vi "Parse Controls and Indicators.vi"(8 "Error In":errorcluster, 9 "Indicators":T1[](array[typedef]), 11 "Controls":T1[](array[typedef])) -> (0 "Error Out":errorcluster, 2 "Indicators  Wiki Syntax":string, 3 "Contorls Wiki Syntax":string)   [LabVIEW 2014]
uses:
  Control Info.ctl
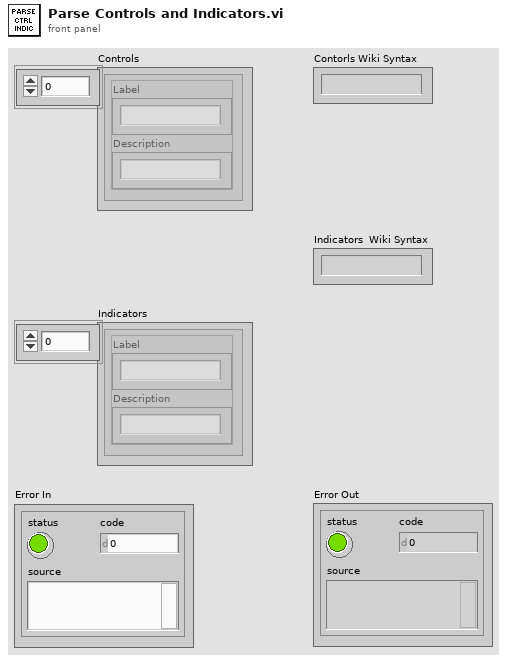
[diagram p1: front panel]
types:
  T1 = typedef "Control Info.ctl" = cluster{"Label":string, "Description":string}
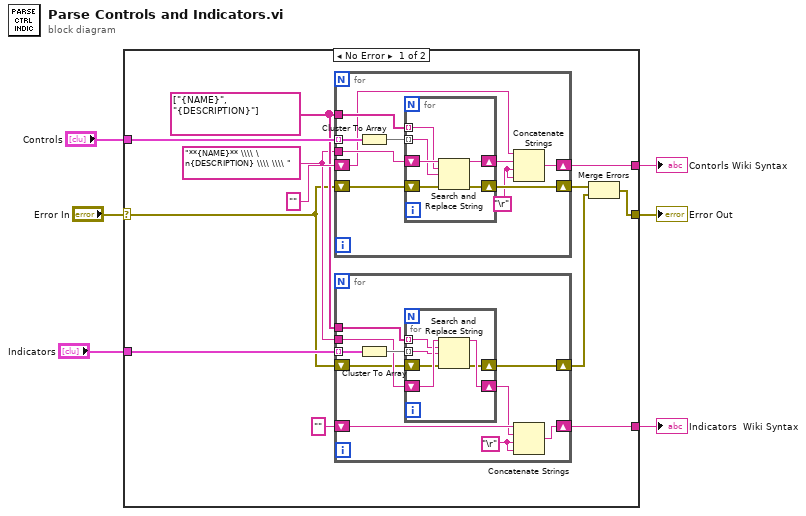
[diagram p0: block diagram]
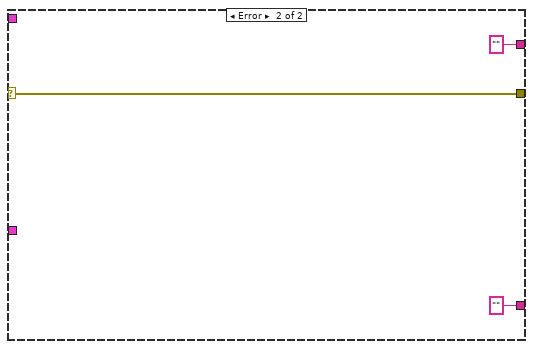
[diagram p2: hidden frame]
diagram:
  n1 = case shown="No Error" "Error In" {
    selector: "Error In" -> [w8 w51]
    tunnel: "Controls" -> [w17 _]
    tunnel: [w16 w51] -> w5
    tunnel: [w15 ""] -> w4
    tunnel: [w14 ""] -> w3
    tunnel: "Indicators" -> [w10 _]
    frame No Error {
      w11 = string[] ["{NAME}", "{DESCRIPTION}"]
      w9 = "**{NAME}** \\\\ \n{DESCRIPTION} \\\\ \\\\ "
      n2 = for {
        tunnel: w17 -> [w44] mode=indexing
        tunnel: w9 -> [w42]
        tunnel: w11 -> [w41]
        shift-right: [w39] -> w13
        shift-left: w8 -> [w40]
        shift-right: [w36] -> w14
        shift-left: "" -> [w38]
        w35 = "\r"
        n3 = Cluster To Array(cluster=w44) -> (array=w43:string[])
        n4 = for {
          tunnel: w43 -> [w47] mode=indexing
          shift-right: [w49] -> w37
          shift-left: w42 -> [w50]
          tunnel: w41 -> [w48] mode=indexing
          shift-right: [w45] -> w39
          shift-left: w40 -> [w46]
          n5 = Search and Replace String(input string=w50, search string=w48, replace string=w47, error in=w46) -> (result string=w49:string, error out=w45:errorcluster)  [unwired: 4 in, 2 out]
        }
        n6 = Concatenate Strings(w38, w37, w35, w35) -> (w36:string)
      }
      n7 = for {
        tunnel: w10 -> [w28] mode=indexing
        tunnel: w9 -> [w26]
        tunnel: w11 -> [w25]
        shift-right: [w23] -> w12
        shift-left: w8 -> [w24]
        shift-right: [w20] -> w15
        shift-left: "" -> [w22]
        w19 = "\r"
        n8 = Cluster To Array(cluster=w28) -> (array=w27:string[])
        n9 = for {
          tunnel: w27 -> [w31] mode=indexing
          shift-right: [w33] -> w21
          shift-left: w26 -> [w34]
          tunnel: w25 -> [w32] mode=indexing
          shift-right: [w29] -> w23
          shift-left: w24 -> [w30]
          n10 = Search and Replace String(input string=w34, search string=w32, replace string=w31, error in=w30) -> (result string=w33:string, error out=w29:errorcluster)  [unwired: 4 in, 2 out]
        }
        n11 = Concatenate Strings(w22, w21, w19, w19) -> (w20:string)
      }
      n12 = Merge Errors(w13, w12) -> (w16:errorcluster)
    }
    frame Error {
    }
  }
  "Error Out" <- w5
  "Indicators  Wiki Syntax" <- w4
  "Contorls Wiki Syntax" <- w3
